vi "compute success rate.vi"(9 "shift index":i32, 10 "output array":i8[](array[numeric]), 11 "input array":i8[](array[numeric])) -> (3 "Bitwise success rate":dbl)   [LabVIEW 2013]
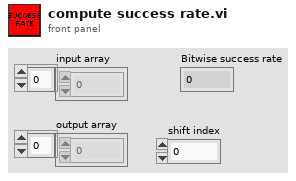
[diagram p1: front panel]
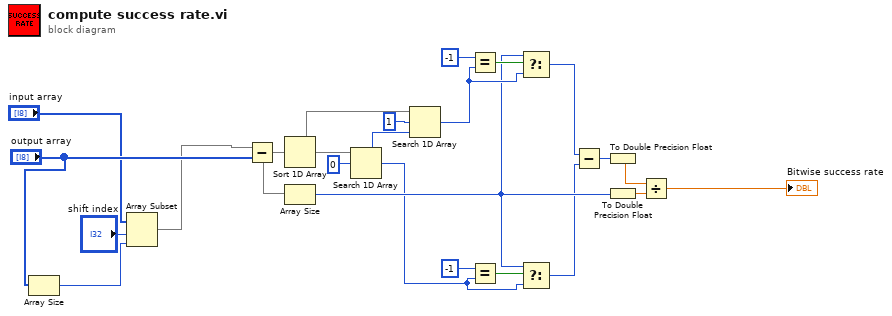
[diagram p0: block diagram]
diagram:
  n1 = Array Size(array="output array") -> (size(s)=w4:i32)
  n2 = Array Subset(array="input array", index="shift index", length=w4) -> (w1:i8[])
  n3 = Subtract(x=w1, y="output array") -> (x-y=w22:i8[])
  n4 = Sort 1D Array(array=w22) -> (sorted array=w16:i8[])
  n5 = Array Size(array=w22) -> (size(s)=w8:i32)
  n6 = Search 1D Array(1D array=w16, element=i8 0) -> (index of element=w7:i32)  [unwired: 1 in]
  n7 = Search 1D Array(1D array=w16, element=i8 1, start index (0)=w7) -> (index of element=w12:i32)
  n8 = Equal?(x=-1, y=w12) -> (x = y?=w13:bool)
  n9 = Equal?(x=-1, y=w7) -> (x = y?=w10:bool)
  n10 = Select(t=w8, s=w13, f=w12) -> (s? t:f=w11:i32)
  n11 = Select(t=w8, s=w10, f=w7) -> (s? t:f=w6:i32)
  n12 = Subtract(x=w11, y=w6) -> (x-y=w18:i32)
  n13 = To Double Precision Float(number=w18) -> (double precision float=w21:dbl)
  n14 = To Double Precision Float(number=w8) -> (double precision float=w20:dbl)
  n15 = Divide(x=w21, y=w20) -> (x/y=→"Bitwise success rate":dbl)
